vi "Mining Setup.vi"() -> (3 "output cluster":T3)   [LabVIEW 2012]
uses:
  <vilib>/vision/Image Controls.llb/IMAQ Image.ctl
  <vilib>/httpClient/ClientHandle.ctl
  <vilib>/httpClient/LabVIEWHTTPClient.lvlib
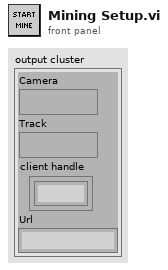
[diagram p1: front panel]
types:
  T1 = typedef "IMAQ Image.ctl" = refnum<image>
  T2 = typedef "LabVIEWHTTPClient.lvlib/ClientHandle.ctl" = refnum<k1>
  T3 = cluster{"Camera":T1, "Track":T1, "client handle":T2, "Url":string}
  T4 = typedef "Image Type" = u32
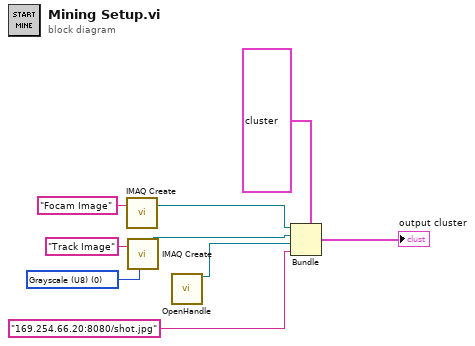
[diagram p0: block diagram]
diagram:
  w7 = T4 0 items=["Grayscale (U8)", "Grayscale (I16)", "Grayscale (SGL)", "Complex (CSG)", "RGB (U32)", "HSL (U32)", "RGB (U64)", "Grayscale (U16)"] ("Image Type")
  n1 = call "IMAQ Create"("Image Name"="Focam Image") -> ("New Image"=w5:T1)  [unwired: 4 in, 1 out]
  n2 = call "IMAQ Create"("Image Name"="Track Image", "Image Type"=w7) -> ("New Image"=w6:T1)  [unwired: 3 in, 1 out]
  n3 = call <vilib>:"OpenHandle.vi"() -> ("client handle out"=w3:T2)  [unwired: 14 in, 1 out]
  n4 = Bundle(cluster=T3 {"Camera"=refnum, "Track"=refnum, "client handle"=refnum, "Url"=""}, "Camera"=w5, "Track"=w6, "client handle"=w3, "Url"="169.254.66.20:8080/shot.jpg") -> (→"output cluster":T3)
